vi "Check_Module_Information.vi"(0 "Address Cluster":T1 {"PCU_communcation_method" items=["GPIB", "C232C", "TCPIP", "USB"]; "tsl_communcation_method" items=["GPIB", "C232C", "TCPIP", "USB"]; "MPM_communcation_method" items=["GPIB", "C232C", "TCPIP", "USB"]}, 11 "错误输入（无错误）":errorcluster caption="error in") -> (4 "Address Cluster out":T1 {"PCU_communcation_method" items=["GPIB", "C232C", "TCPIP", "USB"]; "tsl_communcation_method" items=["GPIB", "C232C", "TCPIP", "USB"]; "MPM_communcation_method" items=["GPIB", "C232C", "TCPIP", "USB"]}, 6 "Flag_215":bool, 8 "Flag_211":bool, 10 "Flag_213":bool, 15 "error out":errorcluster)   [LabVIEW 2017]
doc: "check Module information inside system"
uses:
  CTL/Address Cluster.ctl
  D:/test/PDLSTS/LV_PDL LvVer17.0/LV_PDL_x64/DLL/InstrumentDLL.dll
  DLL/InstrumentDLL.dll
  Share/MPM_PowerMonitorType.vi
panel:
  in  "counter_215":i32
  in  "enable_module_count":i32
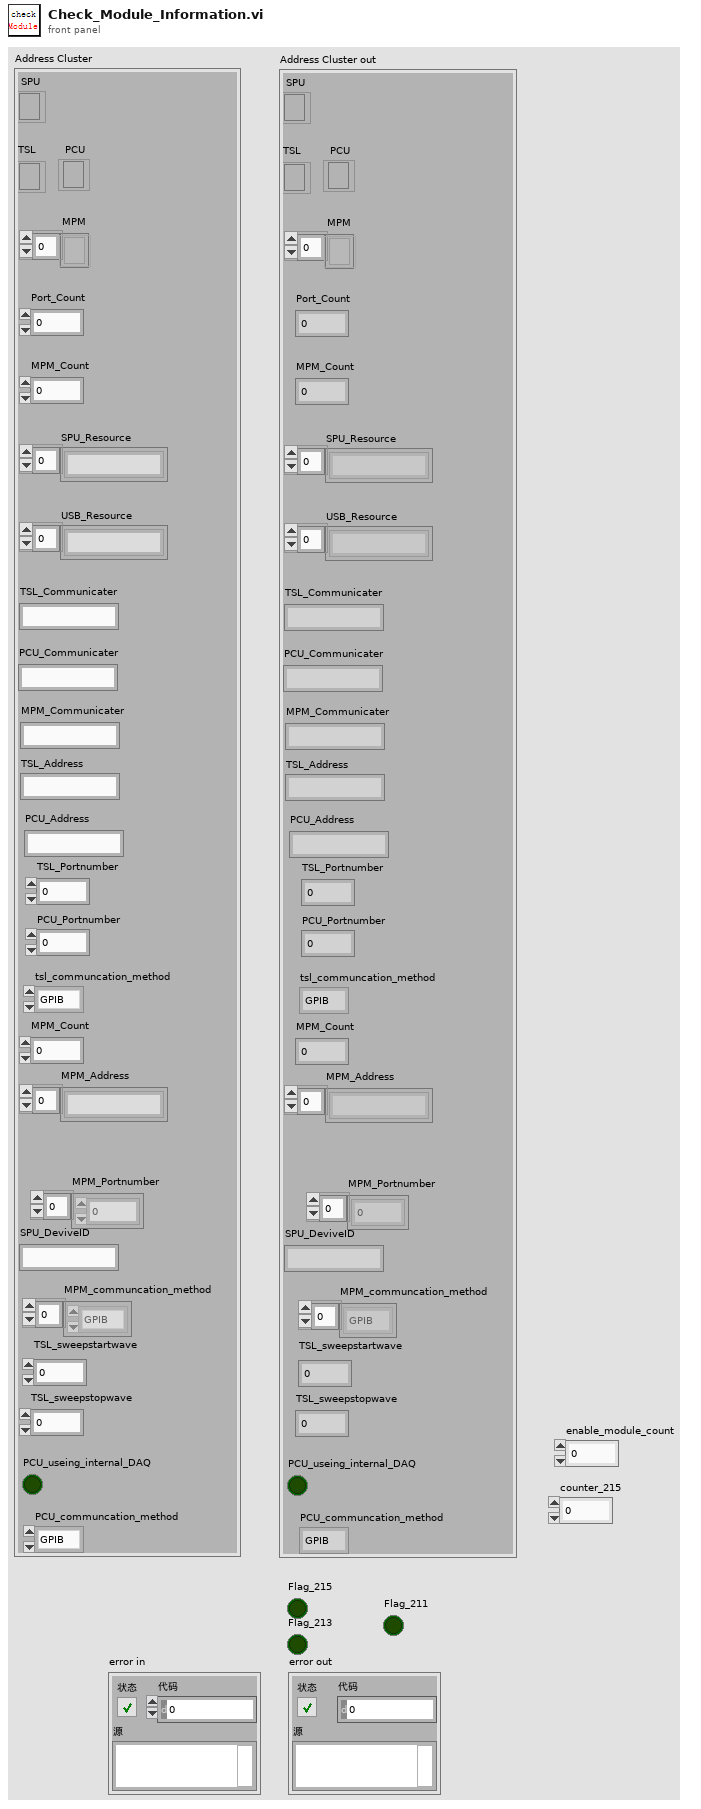
[diagram p1: front panel]
types:
  T1 = typedef "Address Cluster.ctl" = cluster{"SPU":refnum<k24>, "MPM":refnum<k24>[], "Port_Count":dbl, "MPM_Count":dbl, "SPU_Resource":string[], "USB_Resource":string[], "MPM_Communicater":string, "MPM_Count":dbl, "MPM_Address":string[], "MPM_Portnumber":dbl[], "SPU_DeviveID":string, "MPM_communcation_method":i32[], "TSL_sweepstartwave":dbl, "TSL_sweepstopwave":dbl, "TSL_Address":string, "TSL_Communicater":string, "TSL":refnum<k24>, "tsl_communcation_method":i32, "TSL_Portnumber":dbl, "PCU":refnum<k24>, "PCU_Communicater":string, "PCU_Address":string, "PCU_Portnumber":dbl, "PCU_useing_internal_DAQ":bool, "PCU_communcation_method":i32}
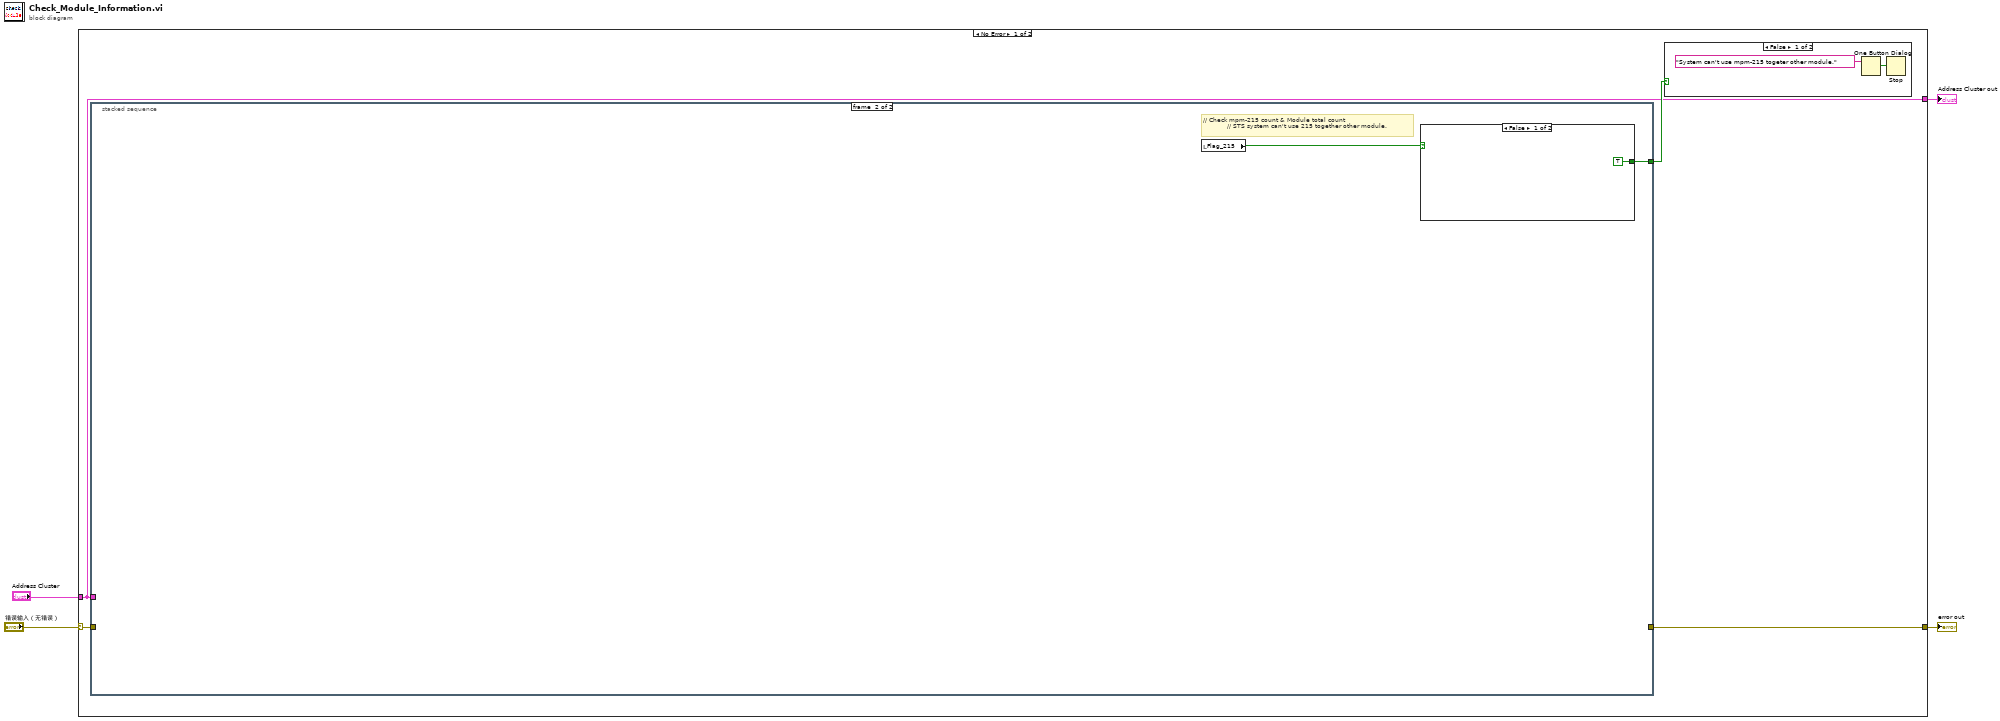
[diagram p0: block diagram]
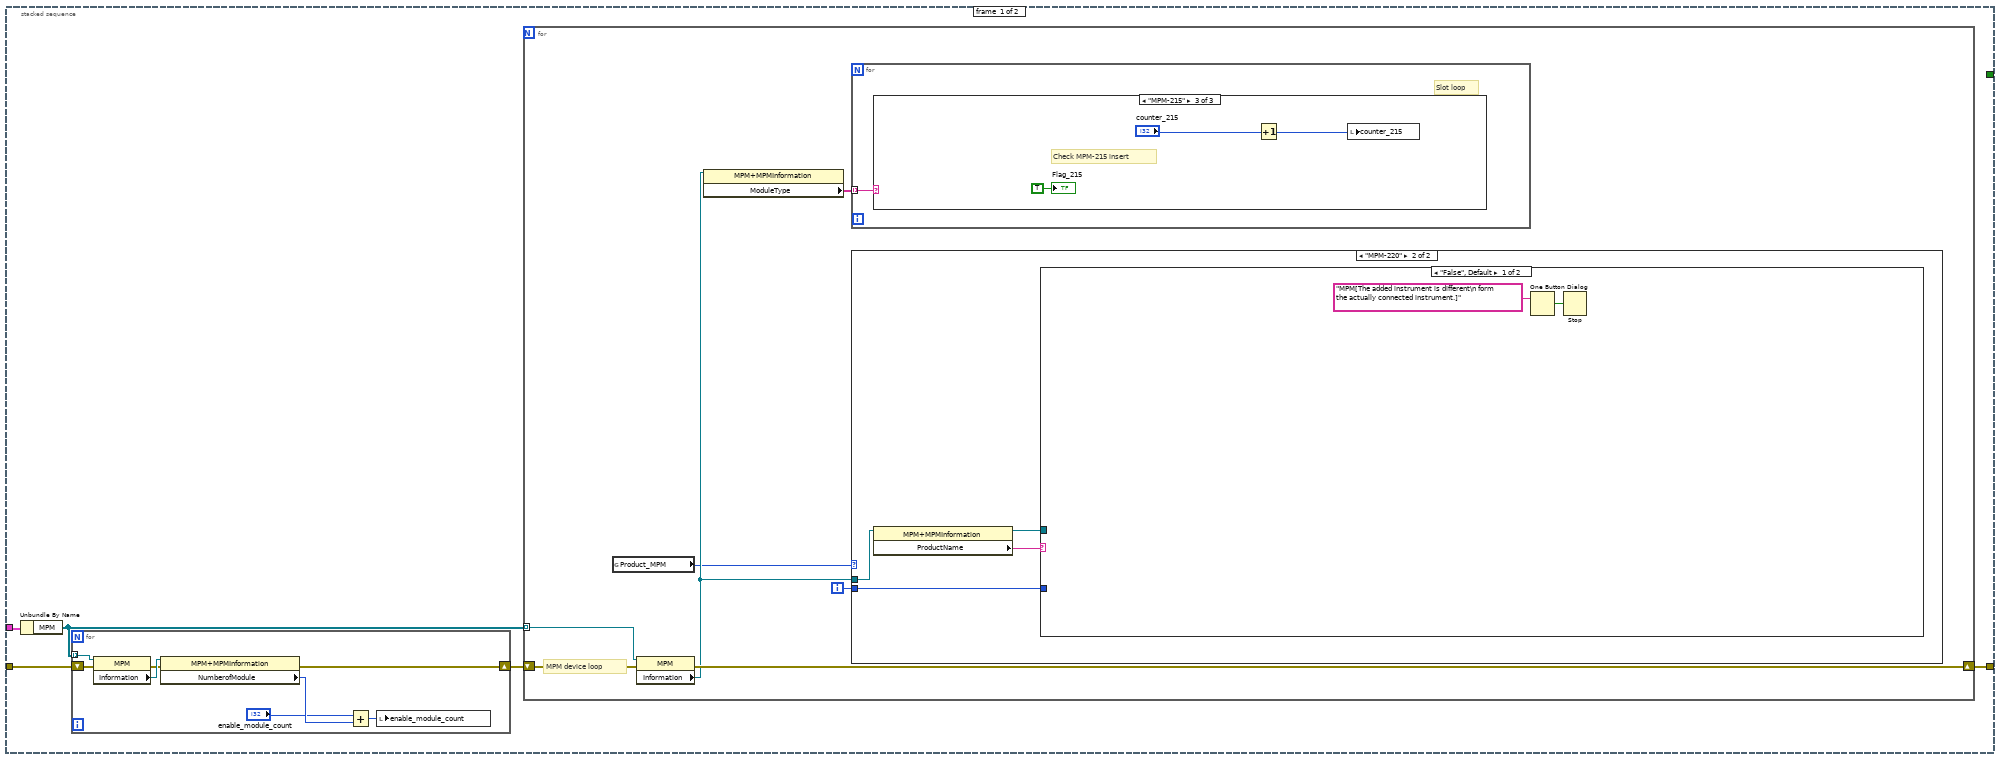
[diagram p3: hidden frame]
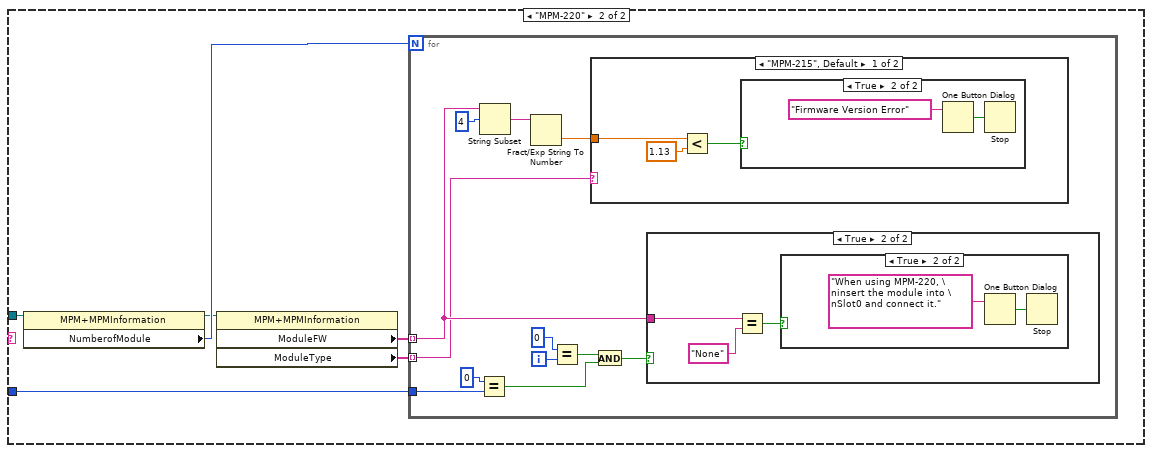
[diagram p5: hidden frame]
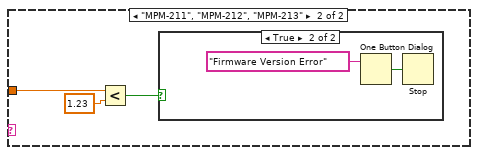
[diagram p7: hidden frame]
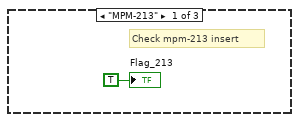
[diagram p11: hidden frame]
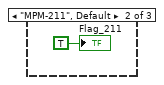
[diagram p12: hidden frame]
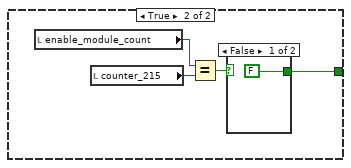
[diagram p13: hidden frame]
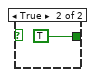
[diagram p14: hidden frame]
diagram:
  n1 = case shown="No Error" "错误输入（无错误）" {
    selector: "错误输入（无错误）" -> [w7 w86]
    tunnel: "Address Cluster" -> [w5 w85]
    tunnel: [w6 w86] -> w2
    tunnel: [w5 w85] -> w1
    frame No Error {
      n2 = stacked-sequence {
        tunnel: w5 -> [w15 _]
        tunnel: [_ w76] -> w8
        tunnel: w7 -> [w13 _]
        tunnel: [w11 _] -> w6
        frame #0 {
          n3 = Unbundle By Name(w15) -> ("MPM"=w14:refnum<k24>[])
          n4 = for {
            tunnel: w14 -> [w23] mode=indexing
            shift-right: [w16] -> w12
            shift-left: w13 -> [w18]
            n5 = property on="属性节点" class="MPM"(reference=w23, error in=w18) -> (error out=w17:errorcluster, "Information"=w22:refnum<k24>)  [unwired: 1 out]
            n6 = property class="MPM+MPMInformation"(reference=w22, error in=w17) -> (error out=w16:errorcluster, "NumberofModule"=w21:i32)  [unwired: 1 out]
            n7 = Add(x="enable_module_count", y=w21) -> (x+y=w19:i32)
            n8 = local write "enable_module_count"(w19) -> ()
          }
          n9 = for {
            tunnel: w14 -> [w30] mode=indexing
            shift-right: [w27] -> w11
            shift-left: w12 -> [w28]
            i -> [w25]
            # "MPM device loop"
            n10 = global read "MPM_PowerMonitorType.vi" "Product_MPM"() -> (w24:enum32{"MPM-210/210H", "MPM-220"})
            n11 = property on="属性节点" class="MPM"(reference=w30, error in=w28) -> (error out=w27:errorcluster, "Information"=w26:refnum<k24>)  [unwired: 1 out]
            n12 = property class="MPM+MPMInformation"(reference=w26) -> ("ModuleType"=w29:string[])  [unwired: 1 in, 2 out]
            n13 = for {
              tunnel: w29 -> [w70] mode=indexing
              # "Slot loop"
              n14 = case shown="\"MPM-215\"" w70 {
                frame "MPM-213" {
                  # "Check mpm-213 insert"
                  "Flag_213" <- TRUE ("Flag_213")
                }
                frame "MPM-211", Default {
                  "Flag_211" <- TRUE ("Flag_213")
                }
                frame "MPM-215" {
                  # "Check MPM-215 insert"
                  n15 = Increment(x="counter_215") -> (x+1=w73:i32)
                  n16 = local write "counter_215"(w73) -> ()
                  "Flag_215" <- TRUE ("Flag_215")
                }
              }
            }
            n17 = case shown="\"MPM-220\"" w24 {
              tunnel: w26 -> [_ w34]
              tunnel: w25 -> [_ w31]
              frame "MPM-210/210H", Default {
              }
              frame "MPM-220" {
                n18 = property class="MPM+MPMInformation"(reference=w34) -> (reference out=w32:refnum<k24>, "ProductName"=w33:string)  [unwired: 1 in, 1 out]
                n19 = case shown="\"False\", Default" w33 {
                  tunnel: w32 -> [_ w42]
                  tunnel: w31 -> [_ w40]
                  frame "False", Default {
                    n20 = One Button Dialog(message="MPM[The added instrument is different\n form the actually connected instrument.]") -> (true=w35:bool)  [unwired: 1 in]
                    n21 = Stop(stop? (T)=w35) -> ()
                  }
                  frame "MPM-220" {
                    n22 = property class="MPM+MPMInformation"(reference=w42) -> (reference out=w39:refnum<k24>, "NumberofModule"=w41:i32)  [unwired: 1 in, 1 out]
                    n23 = property class="MPM+MPMInformation"(reference=w39) -> ("ModuleFW"=w38:string[], "ModuleType"=w37:string[])  [unwired: 1 in, 2 out]
                    n24 = for {
                      N: w41 -> [_]
                      tunnel: w40 -> [w54]
                      tunnel: w38 -> [w47] mode=indexing
                      tunnel: w37 -> [w45] mode=indexing
                      i -> [w50]
                      n25 = Equal?(x=0, y=w54) -> (x = y?=w52:bool)
                      n26 = String Subset(string=w47, offset (0)=4) -> (substring=w44:string)  [unwired: 1 in]
                      n27 = Fract/Exp String To Number(string=w44) -> (number=w43:dbl)  [unwired: 3 in, 1 out]
                      n28 = Equal?(x=0, y=w50) -> (x = y?=w49:bool)
                      n29 = case shown="\"MPM-215\", Default" w45 {
                        tunnel: w43 -> [w57 w60]
                        frame "MPM-215", Default {
                          n30 = Less?(x=w57, y=1.13) -> (x < y?=w55:bool)
                          n31 = case shown="True" w55 {
                            frame False {
                            }
                            frame True {
                              n32 = One Button Dialog(message="Firmware Version Error") -> (true=w58:bool)  [unwired: 1 in]
                              n33 = Stop(stop? (T)=w58) -> ()
                            }
                          }
                        }
                        frame "MPM-211", "MPM-212", "MPM-213" {
                          n34 = Less?(x=w60, y=1.23) -> (x < y?=w61:bool)
                          n35 = case shown="True" w61 {
                            frame False {
                            }
                            frame True {
                              n36 = One Button Dialog(message="Firmware Version Error") -> (true=w63:bool)  [unwired: 1 in]
                              n37 = Stop(stop? (T)=w63) -> ()
                            }
                          }
                        }
                      }
                      n38 = And(x=w49, y=w52) -> (x .and. y?=w48:bool)
                      n39 = case shown="True" w48 {
                        tunnel: w47 -> [_ w67]
                        frame False {
                        }
                        frame True {
                          n40 = Equal?(x=w67, y="None") -> (x = y?=w65:bool)
                          n41 = case shown="True" w65 {
                            frame False {
                            }
                            frame True {
                              n42 = One Button Dialog(message="When using MPM-220, \ninsert the module into \nSlot0 and connect it.") -> (true=w68:bool)  [unwired: 1 in]
                              n43 = Stop(stop? (T)=w68) -> ()
                            }
                          }
                        }
                      }
                    }
                  }
                }
              }
            }
          }
        }
        frame #1 {
          # "// Check mpm-215 count & Module total count\n            // STS system can't use 215 together other module."
          n44 = local read "Flag_215"() -> (w77:bool)
          n45 = case shown="False" w77 {
            tunnel: [TRUE w79] -> w76
            frame False {
            }
            frame True {
              n46 = local read "enable_module_count"() -> (w82:i32)
              n47 = local read "counter_215"() -> (w81:i32)
              n48 = Equal?(x=w82, y=w81) -> (x = y?=w80:bool)
              n49 = case shown="False" w80 {
                tunnel: [FALSE TRUE] -> w79
                frame False {
                }
                frame True {
                }
              }
            }
          }
        }
      }
      n50 = case shown="False" w8 {
        frame False {
          n51 = One Button Dialog(message="System can't use mpm-215 togeter other module." ("消息")) -> (true=w9:bool)  [unwired: 1 in]
          n52 = Stop(stop? (T)=w9) -> ()
        }
        frame True {
        }
      }
    }
    frame Error {
    }
  }
  "Address Cluster out" <- w1
  "error out" <- w2
